vi "Manual control operator action.vi"(6 "error in":errorcluster, 8 "Abort Test":T1, 9 "Motion Steps in":string[](array[string]), 11 "input cluster":T2={"AT glass position"={"Tag Name"="S060.PXI.Signals.PlltData.SN", "Network Path"="172.15.51.1,1,0", "use opc"=FALSE, "DataSocket Reference"={"CWDSLib._DCWDataSocket"=refnum, "CWDSLib._DCWData"=refnum, "OnDataUpdated"=0, "OnStatusUpdated"=0}}, "AT shade position"={"Tag Name"="S060.PXI.Signals.PlltData.SN", "Network Path"="172.15.51.1,1,0", "use opc"=FALSE, "DataSocket Reference"={"CWDSLib._DCWDataSocket"=refnum, "CWDSLib._DCWData"=refnum, "OnDataUpdated"=0, "OnStatusUpdated"=0}}, "AT in glass wand lower pos"={"Tag Name"="S060.PXI.Signals.PlltData.SN", "Network Path"="172.15.51.1,1,0", "use opc"=FALSE, "DataSocket Reference"={"CWDSLib._DCWDataSocket"=refnum, "CWDSLib._DCWData"=refnum, "OnDataUpdated"=0, "OnStatusUpdated"=0}}, "AT in glass wand up pos"={"Tag Name"="S060.PXI.Signals.PlltData.SN", "Network Path"="172.15.51.1,1,0", "use opc"=FALSE, "DataSocket Reference"={"CWDSLib._DCWDataSocket"=refnum, "CWDSLib._DCWData"=refnum, "OnDataUpdated"=0, "OnStatusUpdated"=0}}, "AT in sunshad wand lower pos"={"Tag Name"="S060.PXI.Signals.PlltData.SN", "Network Path"="172.15.51.1,1,0", "use opc"=FALSE, "DataSocket Reference"={"CWDSLib._DCWDataSocket"=refnum, "CWDSLib._DCWData"=refnum, "OnDataUpdated"=0, "OnStatusUpdated"=0}}, "AT in sunshad wand up pos"={"Tag Name"="S060.PXI.Signals.PlltData.SN", "Network Path"="172.15.51.1,1,0", "use opc"=FALSE, "DataSocket Reference"={"CWDSLib._DCWDataSocket"=refnum, "CWDSLib._DCWData"=refnum, "OnDataUpdated"=0, "OnStatusUpdated"=0}}, "AT in wand home pos"={"Tag Name"="S060.PXI.Signals.PlltData.SN", "Network Path"="172.15.51.1,1,0", "use opc"=FALSE, "DataSocket Reference"={"CWDSLib._DCWDataSocket"=refnum, "CWDSLib._DCWData"=refnum, "OnDataUpdated"=0, "OnStatusUpdated"=0}}, "LVDT's Extended"={"Tag Name"="S060.PXI.Signals.PlltData.SN", "Network Path"="172.15.51.1,1,0", "use opc"=FALSE, "DataSocket Reference"={"CWDSLib._DCWDataSocket"=refnum, "CWDSLib._DCWData"=refnum, "OnDataUpdated"=0, "OnStatusUpdated"=0}}, "bolt check 1"={"Tag Name"="S060.PXI.Signals.PlltData.SN", "Network Path"="172.15.51.1,1,0", "use opc"=FALSE, "DataSocket Reference"={"CWDSLib._DCWDataSocket"=refnum, "CWDSLib._DCWData"=refnum, "OnDataUpdated"=0, "OnStatusUpdated"=0}}, "bolt check 2"={"Tag Name"="S060.PXI.Signals.PlltData.SN", "Network Path"="172.15.51.1,1,0", "use opc"=FALSE, "DataSocket Reference"={"CWDSLib._DCWDataSocket"=refnum, "CWDSLib._DCWData"=refnum, "OnDataUpdated"=0, "OnStatusUpdated"=0}}, "bolt check 3"={"Tag Name"="S060.PXI.Signals.PlltData.SN", "Network Path"="172.15.51.1,1,0", "use opc"=FALSE, "DataSocket Reference"={"CWDSLib._DCWDataSocket"=refnum, "CWDSLib._DCWData"=refnum, "OnDataUpdated"=0, "OnStatusUpdated"=0}}, "bolt check 4"={"Tag Name"="S060.PXI.Signals.PlltData.SN", "Network Path"="172.15.51.1,1,0", "use opc"=FALSE, "DataSocket Reference"={"CWDSLib._DCWDataSocket"=refnum, "CWDSLib._DCWData"=refnum, "OnDataUpdated"=0, "OnStatusUpdated"=0}}, "bolt check 5"={"Tag Name"="S060.PXI.Signals.PlltData.SN", "Network Path"="172.15.51.1,1,0", "use opc"=FALSE, "DataSocket Reference"={"CWDSLib._DCWDataSocket"=refnum, "CWDSLib._DCWData"=refnum, "OnDataUpdated"=0, "OnStatusUpdated"=0}}, "bolt check 6"={"Tag Name"="S060.PXI.Signals.PlltData.SN", "Network Path"="172.15.51.1,1,0", "use opc"=FALSE, "DataSocket Reference"={"CWDSLib._DCWDataSocket"=refnum, "CWDSLib._DCWData"=refnum, "OnDataUpdated"=0, "OnStatusUpdated"=0}}, "bolt check 7"={"Tag Name"="S060.PXI.Signals.PlltData.SN", "Network Path"="172.15.51.1,1,0", "use opc"=FALSE, "DataSocket Reference"={"CWDSLib._DCWDataSocket"=refnum, "CWDSLib._DCWData"=refnum, "OnDataUpdated"=0, "OnStatusUpdated"=0}}, "bolt check 8"={"Tag Name"="S060.PXI.Signals.PlltData.SN", "Network Path"="172.15.51.1,1,0", "use opc"=FALSE, "DataSocket Reference"={"CWDSLib._DCWDataSocket"=refnum, "CWDSLib._DCWData"=refnum, "OnDataUpdated"=0, "OnStatusUpdated"=0}}, "start"={"Tag Name"="S060.PXI.Signals.PlltData.SN", "Network Path"="172.15.51.1,1,0", "use opc"=FALSE, "DataSocket Reference"={"CWDSLib._DCWDataSocket"=refnum, "CWDSLib._DCWData"=refnum, "OnDataUpdated"=0, "OnStatusUpdated"=0}}, "abort"={"Tag Name"="S060.PXI.Signals.PlltData.SN", "Network Path"="172.15.51.1,1,0", "use opc"=FALSE, "DataSocket Reference"={"CWDSLib._DCWDataSocket"=refnum, "CWDSLib._DCWData"=refnum, "OnDataUpdated"=0, "OnStatusUpdated"=0}}, "LVDT's Retracted"={"Tag Name"="S060.PXI.Signals.PlltData.SN", "Network Path"="172.15.51.1,1,0", "use opc"=FALSE, "DataSocket Reference"={"CWDSLib._DCWDataSocket"=refnum, "CWDSLib._DCWData"=refnum, "OnDataUpdated"=0, "OnStatusUpdated"=0}}, "manual barcode print"={"Tag Name"="S060.PXI.Signals.PlltData.SN", "Network Path"="172.15.51.1,1,0", "use opc"=FALSE, "DataSocket Reference"={"CWDSLib._DCWDataSocket"=refnum, "CWDSLib._DCWData"=refnum, "OnDataUpdated"=0, "OnStatusUpdated"=0}}, "ss servo at open"={"Tag Name"="S060.PXI.Signals.PlltData.SN", "Network Path"="172.15.51.1,1,0", "use opc"=FALSE, "DataSocket Reference"={"CWDSLib._DCWDataSocket"=refnum, "CWDSLib._DCWData"=refnum, "OnDataUpdated"=0, "OnStatusUpdated"=0}}, "ss servo at close"={"Tag Name"="S060.PXI.Signals.PlltData.SN", "Network Path"="172.15.51.1,1,0", "use opc"=FALSE, "DataSocket Reference"={"CWDSLib._DCWDataSocket"=refnum, "CWDSLib._DCWData"=refnum, "OnDataUpdated"=0, "OnStatusUpdated"=0}}, "ss servo opening"={"Tag Name"="S060.PXI.Signals.PlltData.SN", "Network Path"="172.15.51.1,1,0", "use opc"=FALSE, "DataSocket Reference"={"CWDSLib._DCWDataSocket"=refnum, "CWDSLib._DCWData"=refnum, "OnDataUpdated"=0, "OnStatusUpdated"=0}}, "ss servo closing"={"Tag Name"="S060.PXI.Signals.PlltData.SN", "Network Path"="172.15.51.1,1,0", "use opc"=FALSE, "DataSocket Reference"={"CWDSLib._DCWDataSocket"=refnum, "CWDSLib._DCWData"=refnum, "OnDataUpdated"=0, "OnStatusUpdated"=0}}, "control slide at home"={"Tag Name"="S060.PXI.Signals.PlltData.SN", "Network Path"="172.15.51.1,1,0", "use opc"=FALSE, "DataSocket Reference"={"CWDSLib._DCWDataSocket"=refnum, "CWDSLib._DCWData"=refnum, "OnDataUpdated"=0, "OnStatusUpdated"=0}}, "control slide left good"={"Tag Name"="S060.PXI.Signals.PlltData.SN", "Network Path"="172.15.51.1,1,0", "use opc"=FALSE, "DataSocket Reference"={"CWDSLib._DCWDataSocket"=refnum, "CWDSLib._DCWData"=refnum, "OnDataUpdated"=0, "OnStatusUpdated"=0}}, "control slide left over stroke"={"Tag Name"="S060.PXI.Signals.PlltData.SN", "Network Path"="172.15.51.1,1,0", "use opc"=FALSE, "DataSocket Reference"={"CWDSLib._DCWDataSocket"=refnum, "CWDSLib._DCWData"=refnum, "OnDataUpdated"=0, "OnStatusUpdated"=0}}, "control slide right good"={"Tag Name"="S060.PXI.Signals.PlltData.SN", "Network Path"="172.15.51.1,1,0", "use opc"=FALSE, "DataSocket Reference"={"CWDSLib._DCWDataSocket"=refnum, "CWDSLib._DCWData"=refnum, "OnDataUpdated"=0, "OnStatusUpdated"=0}}, "control slide right over stroke"={"Tag Name"="S060.PXI.Signals.PlltData.SN", "Network Path"="172.15.51.1,1,0", "use opc"=FALSE, "DataSocket Reference"={"CWDSLib._DCWDataSocket"=refnum, "CWDSLib._DCWData"=refnum, "OnDataUpdated"=0, "OnStatusUpdated"=0}}, "wind deflector high speed pos"={"Tag Name"="S060.PXI.Signals.PlltData.SN", "Network Path"="172.15.51.1,1,0", "use opc"=FALSE, "DataSocket Reference"={"CWDSLib._DCWDataSocket"=refnum, "CWDSLib._DCWData"=refnum, "OnDataUpdated"=0, "OnStatusUpdated"=0}}, "wind deflector low speed pos"={"Tag Name"="S060.PXI.Signals.PlltData.SN", "Network Path"="172.15.51.1,1,0", "use opc"=FALSE, "DataSocket Reference"={"CWDSLib._DCWDataSocket"=refnum, "CWDSLib._DCWData"=refnum, "OnDataUpdated"=0, "OnStatusUpdated"=0}}, "AT VentPMACatHome"={"Tag Name"="S060.PXI.Signals.PlltData.SN", "Network Path"="172.15.51.1,1,0", "use opc"=FALSE, "DataSocket Reference"={"CWDSLib._DCWDataSocket"=refnum, "CWDSLib._DCWData"=refnum, "OnDataUpdated"=0, "OnStatusUpdated"=0}}, "AT VentPMACisExtend"={"Tag Name"="S060.PXI.Signals.PlltData.SN", "Network Path"="172.15.51.1,1,0", "use opc"=FALSE, "DataSocket Reference"={"CWDSLib._DCWDataSocket"=refnum, "CWDSLib._DCWData"=refnum, "OnDataUpdated"=0, "OnStatusUpdated"=0}}, "SS Barcode Scanner Bypassed"={"Tag Name"="S060.PXI.Signals.PlltData.SN", "Network Path"="172.15.51.1,1,0", "use opc"=FALSE, "DataSocket Reference"={"CWDSLib._DCWDataSocket"=refnum, "CWDSLib._DCWData"=refnum, "OnDataUpdated"=0, "OnStatusUpdated"=0}}, "Check Frame Barcode"={"Tag Name"="S060.PXI.Signals.PlltData.SN", "Network Path"="172.15.51.1,1,0", "use opc"=FALSE, "DataSocket Reference"={"CWDSLib._DCWDataSocket"=refnum, "CWDSLib._DCWData"=refnum, "OnDataUpdated"=0, "OnStatusUpdated"=0}}, "Z LVDTs Extended"={"Tag Name"="S060.PXI.Signals.PlltData.SN", "Network Path"="172.15.51.1,1,0", "use opc"=FALSE, "DataSocket Reference"={"CWDSLib._DCWDataSocket"=refnum, "CWDSLib._DCWData"=refnum, "OnDataUpdated"=0, "OnStatusUpdated"=0}}, "NVH Operator Pass"={"Tag Name"="S060.PXI.Signals.PlltData.SN", "Network Path"="172.15.51.1,1,0", "use opc"=FALSE, "DataSocket Reference"={"CWDSLib._DCWDataSocket"=refnum, "CWDSLib._DCWData"=refnum, "OnDataUpdated"=0, "OnStatusUpdated"=0}}, "NVH Operator Fail"={"Tag Name"="S060.PXI.Signals.PlltData.SN", "Network Path"="172.15.51.1,1,0", "use opc"=FALSE, "DataSocket Reference"={"CWDSLib._DCWDataSocket"=refnum, "CWDSLib._DCWData"=refnum, "OnDataUpdated"=0, "OnStatusUpdated"=0}}, "NVH Operator Express Glass Open"={"Tag Name"="S060.PXI.Signals.PlltData.SN", "Network Path"="172.15.51.1,1,0", "use opc"=FALSE, "DataSocket Reference"={"CWDSLib._DCWDataSocket"=refnum, "CWDSLib._DCWData"=refnum, "OnDataUpdated"=0, "OnStatusUpdated"=0}}, "NVH Operator Express Glass Close"={"Tag Name"="S060.PXI.Signals.PlltData.SN", "Network Path"="172.15.51.1,1,0", "use opc"=FALSE, "DataSocket Reference"={"CWDSLib._DCWDataSocket"=refnum, "CWDSLib._DCWData"=refnum, "OnDataUpdated"=0, "OnStatusUpdated"=0}}, "NVH Operator Express Rollo Open01"={"Tag Name"="S060.PXI.Signals.PlltData.SN", "Network Path"="172.15.51.1,1,0", "use opc"=FALSE, "DataSocket Reference"={"CWDSLib._DCWDataSocket"=refnum, "CWDSLib._DCWData"=refnum, "OnDataUpdated"=0, "OnStatusUpdated"=0}}, "NVH Operator Express Rollo Close01"={"Tag Name"="S060.PXI.Signals.PlltData.SN", "Network Path"="172.15.51.1,1,0", "use opc"=FALSE, "DataSocket Reference"={"CWDSLib._DCWDataSocket"=refnum, "CWDSLib._DCWData"=refnum, "OnDataUpdated"=0, "OnStatusUpdated"=0}}, "NVH Operator Express Rollo Open02"={"Tag Name"="S060.PXI.Signals.PlltData.SN", "Network Path"="172.15.51.1,1,0", "use opc"=FALSE, "DataSocket Reference"={"CWDSLib._DCWDataSocket"=refnum, "CWDSLib._DCWData"=refnum, "OnDataUpdated"=0, "OnStatusUpdated"=0}}, "NVH Operator Express Rollo Close02"={"Tag Name"="S060.PXI.Signals.PlltData.SN", "Network Path"="172.15.51.1,1,0", "use opc"=FALSE, "DataSocket Reference"={"CWDSLib._DCWDataSocket"=refnum, "CWDSLib._DCWData"=refnum, "OnDataUpdated"=0, "OnStatusUpdated"=0}}, "NVH Operator Vent Open Noise"={"Tag Name"="S060.PXI.Signals.PlltData.SN", "Network Path"="172.15.51.1,1,0", "use opc"=FALSE, "DataSocket Reference"={"CWDSLib._DCWDataSocket"=refnum, "CWDSLib._DCWData"=refnum, "OnDataUpdated"=0, "OnStatusUpdated"=0}}, "NVH Operator Vent Close Noise"={"Tag Name"="S060.PXI.Signals.PlltData.SN", "Network Path"="172.15.51.1,1,0", "use opc"=FALSE, "DataSocket Reference"={"CWDSLib._DCWDataSocket"=refnum, "CWDSLib._DCWData"=refnum, "OnDataUpdated"=0, "OnStatusUpdated"=0}}, "NVH Operator Sunshade Open Noise"={"Tag Name"="S060.PXI.Signals.PlltData.SN", "Network Path"="172.15.51.1,1,0", "use opc"=FALSE, "DataSocket Reference"={"CWDSLib._DCWDataSocket"=refnum, "CWDSLib._DCWData"=refnum, "OnDataUpdated"=0, "OnStatusUpdated"=0}}, "NVH Operator Sunshade Close Noise"={"Tag Name"="S060.PXI.Signals.PlltData.SN", "Network Path"="172.15.51.1,1,0", "use opc"=FALSE, "DataSocket Reference"={"CWDSLib._DCWDataSocket"=refnum, "CWDSLib._DCWData"=refnum, "OnDataUpdated"=0, "OnStatusUpdated"=0}}, "NVH Operator Glass Open Noise"={"Tag Name"="S060.PXI.Signals.PlltData.SN", "Network Path"="172.15.51.1,1,0", "use opc"=FALSE, "DataSocket Reference"={"CWDSLib._DCWDataSocket"=refnum, "CWDSLib._DCWData"=refnum, "OnDataUpdated"=0, "OnStatusUpdated"=0}}, "NVH Operator Glass Close Noise"={"Tag Name"="S060.PXI.Signals.PlltData.SN", "Network Path"="172.15.51.1,1,0", "use opc"=FALSE, "DataSocket Reference"={"CWDSLib._DCWDataSocket"=refnum, "CWDSLib._DCWData"=refnum, "OnDataUpdated"=0, "OnStatusUpdated"=0}}, "NVH Operator Finish"={"Tag Name"="S060.PXI.Signals.PlltData.SN", "Network Path"="172.15.51.1,1,0", "use opc"=FALSE, "DataSocket Reference"={"CWDSLib._DCWDataSocket"=refnum, "CWDSLib._DCWData"=refnum, "OnDataUpdated"=0, "OnStatusUpdated"=0}}, "NVH Operator Check"={"Tag Name"="S060.PXI.Signals.PlltData.SN", "Network Path"="172.15.51.1,1,0", "use opc"=FALSE, "DataSocket Reference"={"CWDSLib._DCWDataSocket"=refnum, "CWDSLib._DCWData"=refnum, "OnDataUpdated"=0, "OnStatusUpdated"=0}}, "windproof position"={"Tag Name"="S060.PXI.Signals.PlltData.SN", "Network Path"="172.15.51.1,1,0", "use opc"=FALSE, "DataSocket Reference"={"CWDSLib._DCWDataSocket"=refnum, "CWDSLib._DCWData"=refnum, "OnDataUpdated"=0, "OnStatusUpdated"=0}}, "NVH Operator Express Glass vent Open"={"Tag Name"="S060.PXI.Signals.PlltData.SN", "Network Path"="172.15.51.1,1,0", "use opc"=FALSE, "DataSocket Reference"={"CWDSLib._DCWDataSocket"=refnum, "CWDSLib._DCWData"=refnum, "OnDataUpdated"=0, "OnStatusUpdated"=0}}, "NVH Operator Express Glass Vent Close"={"Tag Name"="S060.PXI.Signals.PlltData.SN", "Network Path"="172.15.51.1,1,0", "use opc"=FALSE, "DataSocket Reference"={"CWDSLib._DCWDataSocket"=refnum, "CWDSLib._DCWData"=refnum, "OnDataUpdated"=0, "OnStatusUpdated"=0}}, "NVH Operator Re-do"={"Tag Name"="S060.PXI.Signals.PlltData.SN", "Network Path"="172.15.51.1,1,0", "use opc"=FALSE, "DataSocket Reference"={"CWDSLib._DCWDataSocket"=refnum, "CWDSLib._DCWData"=refnum, "OnDataUpdated"=0, "OnStatusUpdated"=0}}, "AT at vent ATS test pos"={"Tag Name"="S060.PXI.Signals.PlltData.SN", "Network Path"="172.15.51.1,1,0", "use opc"=FALSE, "DataSocket Reference"={"CWDSLib._DCWDataSocket"=refnum, "CWDSLib._DCWData"=refnum, "OnDataUpdated"=0, "OnStatusUpdated"=0}}, "AT at vent ATS Home pos"={"Tag Name"="S060.PXI.Signals.PlltData.SN", "Network Path"="172.15.51.1,1,0", "use opc"=FALSE, "DataSocket Reference"={"CWDSLib._DCWDataSocket"=refnum, "CWDSLib._DCWData"=refnum, "OnDataUpdated"=0, "OnStatusUpdated"=0}}, "Start Adjust LVDT"={"Tag Name"="S060.PXI.Signals.PlltData.SN", "Network Path"="172.15.51.1,1,0", "use opc"=FALSE, "DataSocket Reference"={"CWDSLib._DCWDataSocket"=refnum, "CWDSLib._DCWData"=refnum, "OnDataUpdated"=0, "OnStatusUpdated"=0}}, "Finish Adjust LVDT"={"Tag Name"="S060.PXI.Signals.PlltData.SN", "Network Path"="172.15.51.1,1,0", "use opc"=FALSE, "DataSocket Reference"={"CWDSLib._DCWDataSocket"=refnum, "CWDSLib._DCWData"=refnum, "OnDataUpdated"=0, "OnStatusUpdated"=0}}} {"AT in sunshad wand up pos"."DataSocket Reference"."OnStatusUpdated" format="%.0x"; "AT in sunshad wand up pos"."DataSocket Reference"."OnDataUpdated" format="%.0x"; "AT in glass wand up pos"."DataSocket Reference"."OnStatusUpdated" format="%.0x"; "AT in glass wand up pos"."DataSocket Reference"."OnDataUpdated" format="%.0x"; "Finish Adjust LVDT"."DataSocket Reference"."OnStatusUpdated" format="%.0x"; "Finish Adjust LVDT"."DataSocket Reference"."OnDataUpdated" format="%.0x"; "Start Adjust LVDT"."DataSocket Reference"."OnStatusUpdated" format="%.0x"; "Start Adjust LVDT"."DataSocket Reference"."OnDataUpdated" format="%.0x"; "AT at vent ATS Home pos"."DataSocket Reference"."OnStatusUpdated" format="%.0x"; "AT at vent ATS Home pos"."DataSocket Reference"."OnDataUpdated" format="%.0x"; "AT at vent ATS test pos"."DataSocket Reference"."OnStatusUpdated" format="%.0x"; "AT at vent ATS test pos"."DataSocket Reference"."OnDataUpdated" format="%.0x"; "NVH Operator Re-do"."DataSocket Reference"."OnStatusUpdated" format="%.0x"; "NVH Operator Re-do"."DataSocket Reference"."OnDataUpdated" format="%.0x"; "NVH Operator Express Glass Vent Close"."DataSocket Reference"."OnStatusUpdated" format="%.0x"; "NVH Operator Express Glass Vent Close"."DataSocket Reference"."OnDataUpdated" format="%.0x"; "NVH Operator Express Glass vent Open"."DataSocket Reference"."OnStatusUpdated" format="%.0x"; "NVH Operator Express Glass vent Open"."DataSocket Reference"."OnDataUpdated" format="%.0x"; "windproof position"."DataSocket Reference"."OnStatusUpdated" format="%.0x"; "windproof position"."DataSocket Reference"."OnDataUpdated" format="%.0x"; "NVH Operator Check"."DataSocket Reference"."OnStatusUpdated" format="%.0x"; "NVH Operator Check"."DataSocket Reference"."OnDataUpdated" format="%.0x"; "NVH Operator Finish"."DataSocket Reference"."OnStatusUpdated" format="%.0x"; "NVH Operator Finish"."DataSocket Reference"."OnDataUpdated" format="%.0x"; "NVH Operator Glass Close Noise"."DataSocket Reference"."OnStatusUpdated" format="%.0x"; "NVH Operator Glass Close Noise"."DataSocket Reference"."OnDataUpdated" format="%.0x"; "NVH Operator Glass Open Noise"."DataSocket Reference"."OnStatusUpdated" format="%.0x"; "NVH Operator Glass Open Noise"."DataSocket Reference"."OnDataUpdated" format="%.0x"; "NVH Operator Sunshade Close Noise"."DataSocket Reference"."OnStatusUpdated" format="%.0x"; "NVH Operator Sunshade Close Noise"."DataSocket Reference"."OnDataUpdated" format="%.0x"; "NVH Operator Sunshade Open Noise"."DataSocket Reference"."OnStatusUpdated" format="%.0x"; "NVH Operator Sunshade Open Noise"."DataSocket Reference"."OnDataUpdated" format="%.0x"; "NVH Operator Vent Close Noise"."DataSocket Reference"."OnStatusUpdated" format="%.0x"; "NVH Operator Vent Close Noise"."DataSocket Reference"."OnDataUpdated" format="%.0x"; "NVH Operator Vent Open Noise"."DataSocket Reference"."OnStatusUpdated" format="%.0x"; "NVH Operator Vent Open Noise"."DataSocket Reference"."OnDataUpdated" format="%.0x"; "NVH Operator Express Rollo Close02"."DataSocket Reference"."OnStatusUpdated" format="%.0x"; "NVH Operator Express Rollo Close02"."DataSocket Reference"."OnDataUpdated" format="%.0x"; "NVH Operator Express Rollo Open02"."DataSocket Reference"."OnStatusUpdated" format="%.0x"; "NVH Operator Express Rollo Open02"."DataSocket Reference"."OnDataUpdated" format="%.0x"; "NVH Operator Express Rollo Close01"."DataSocket Reference"."OnStatusUpdated" format="%.0x"; "NVH Operator Express Rollo Close01"."DataSocket Reference"."OnDataUpdated" format="%.0x"; "NVH Operator Express Rollo Open01"."DataSocket Reference"."OnStatusUpdated" format="%.0x"; "NVH Operator Express Rollo Open01"."DataSocket Reference"."OnDataUpdated" format="%.0x"; "NVH Operator Express Glass Close"."DataSocket Reference"."OnStatusUpdated" format="%.0x"; "NVH Operator Express Glass Close"."DataSocket Reference"."OnDataUpdated" format="%.0x"; "NVH Operator Express Glass Open"."DataSocket Reference"."OnStatusUpdated" format="%.0x"; "NVH Operator Express Glass Open"."DataSocket Reference"."OnDataUpdated" format="%.0x"; "NVH Operator Fail"."DataSocket Reference"."OnStatusUpdated" format="%.0x"; "NVH Operator Fail"."DataSocket Reference"."OnDataUpdated" format="%.0x"; "NVH Operator Pass"."DataSocket Reference"."OnStatusUpdated" format="%.0x"; "NVH Operator Pass"."DataSocket Reference"."OnDataUpdated" format="%.0x"; "Z LVDTs Extended"."DataSocket Reference"."OnStatusUpdated" format="%.0x"; "Z LVDTs Extended"."DataSocket Reference"."OnDataUpdated" format="%.0x"; "Check Frame Barcode"."DataSocket Reference"."OnStatusUpdated" format="%.0x"; "Check Frame Barcode"."DataSocket Reference"."OnDataUpdated" format="%.0x"; "SS Barcode Scanner Bypassed"."DataSocket Reference"."OnStatusUpdated" format="%.0x"; "SS Barcode Scanner Bypassed"."DataSocket Reference"."OnDataUpdated" format="%.0x"; "AT VentPMACisExtend"."DataSocket Reference"."OnStatusUpdated" format="%.0x"; "AT VentPMACisExtend"."DataSocket Reference"."OnDataUpdated" format="%.0x"; "AT VentPMACatHome"."DataSocket Reference"."OnStatusUpdated" format="%.0x"; "AT VentPMACatHome"."DataSocket Reference"."OnDataUpdated" format="%.0x"; "wind deflector low speed pos"."DataSocket Reference"."OnStatusUpdated" format="%.0x"; "wind deflector low speed pos"."DataSocket Reference"."OnDataUpdated" format="%.0x"; "wind deflector high speed pos"."DataSocket Reference"."OnStatusUpdated" format="%.0x"; "wind deflector high speed pos"."DataSocket Reference"."OnDataUpdated" format="%.0x"; "control slide right over stroke"."DataSocket Reference"."OnStatusUpdated" format="%.0x"; "control slide right over stroke"."DataSocket Reference"."OnDataUpdated" format="%.0x"; "control slide right good"."DataSocket Reference"."OnStatusUpdated" format="%.0x"; "control slide right good"."DataSocket Reference"."OnDataUpdated" format="%.0x"; "control slide left over stroke"."DataSocket Reference"."OnStatusUpdated" format="%.0x"; "control slide left over stroke"."DataSocket Reference"."OnDataUpdated" format="%.0x"; "control slide left good"."DataSocket Reference"."OnStatusUpdated" format="%.0x"; "control slide left good"."DataSocket Reference"."OnDataUpdated" format="%.0x"; "control slide at home"."DataSocket Reference"."OnStatusUpdated" format="%.0x"; "control slide at home"."DataSocket Reference"."OnDataUpdated" format="%.0x"; "ss servo closing"."DataSocket Reference"."OnStatusUpdated" format="%.0x"; "ss servo closing"."DataSocket Reference"."OnDataUpdated" format="%.0x"; "ss servo opening"."DataSocket Reference"."OnStatusUpdated" format="%.0x"; "ss servo opening"."DataSocket Reference"."OnDataUpdated" format="%.0x"; "ss servo at close"."DataSocket Reference"."OnStatusUpdated" format="%.0x"; "ss servo at close"."DataSocket Reference"."OnDataUpdated" format="%.0x"; "ss servo at open"."DataSocket Reference"."OnStatusUpdated" format="%.0x"; "ss servo at open"."DataSocket Reference"."OnDataUpdated" format="%.0x"; "manual barcode print"."DataSocket Reference"."OnStatusUpdated" format="%.0x"; "manual barcode print"."DataSocket Reference"."OnDataUpdated" format="%.0x"; "LVDT's Retracted"."DataSocket Reference"."OnStatusUpdated" format="%.0x"; "LVDT's Retracted"."DataSocket Reference"."OnDataUpdated" format="%.0x"; "abort"."DataSocket Reference"."OnStatusUpdated" format="%.0x"; "abort"."DataSocket Reference"."OnDataUpdated" format="%.0x"; "start"."DataSocket Reference"."OnStatusUpdated" format="%.0x"; "start"."DataSocket Reference"."OnDataUpdated" format="%.0x"; "bolt check 8"."DataSocket Reference"."OnStatusUpdated" format="%.0x"; "bolt check 8"."DataSocket Reference"."OnDataUpdated" format="%.0x"; "bolt check 7"."DataSocket Reference"."OnStatusUpdated" format="%.0x"; "bolt check 7"."DataSocket Reference"."OnDataUpdated" format="%.0x"; "bolt check 6"."DataSocket Reference"."OnStatusUpdated" format="%.0x"; "bolt check 6"."DataSocket Reference"."OnDataUpdated" format="%.0x"; "bolt check 5"."DataSocket Reference"."OnStatusUpdated" format="%.0x"; "bolt check 5"."DataSocket Reference"."OnDataUpdated" format="%.0x"; "bolt check 4"."DataSocket Reference"."OnStatusUpdated" format="%.0x"; "bolt check 4"."DataSocket Reference"."OnDataUpdated" format="%.0x"; "bolt check 3"."DataSocket Reference"."OnStatusUpdated" format="%.0x"; "bolt check 3"."DataSocket Reference"."OnDataUpdated" format="%.0x"; "bolt check 2"."DataSocket Reference"."OnStatusUpdated" format="%.0x"; "bolt check 2"."DataSocket Reference"."OnDataUpdated" format="%.0x"; "bolt check 1"."DataSocket Reference"."OnStatusUpdated" format="%.0x"; "bolt check 1"."DataSocket Reference"."OnDataUpdated" format="%.0x"; "LVDT's Extended"."DataSocket Reference"."OnStatusUpdated" format="%.0x"; "LVDT's Extended"."DataSocket Reference"."OnDataUpdated" format="%.0x"; "AT in wand home pos"."DataSocket Reference"."OnStatusUpdated" format="%.0x"; "AT in wand home pos"."DataSocket Reference"."OnDataUpdated" format="%.0x"; "AT in sunshad wand lower pos"."DataSocket Reference"."OnStatusUpdated" format="%.0x"; "AT in sunshad wand lower pos"."DataSocket Reference"."OnDataUpdated" format="%.0x"; "AT in glass wand lower pos"."DataSocket Reference"."OnStatusUpdated" format="%.0x"; "AT in glass wand lower pos"."DataSocket Reference"."OnDataUpdated" format="%.0x"; "AT shade position"."DataSocket Reference"."OnStatusUpdated" format="%.0x"; "AT shade position"."DataSocket Reference"."OnDataUpdated" format="%.0x"; "AT glass position"."DataSocket Reference"."OnStatusUpdated" format="%.0x"; "AT glass position"."DataSocket Reference"."OnDataUpdated" format="%.0x"}) -> (0 "error out":errorcluster, 1 "Step":string, 2 "data string":string, 3 "Motion Steps out":string[](array[string]))   [LabVIEW 2018]
uses:
  02.Type Def's/station plc read boolean tags.ctl
  05.UserVI's/type defs/plc path and tag.ctl
  <vilib>/Platform/dataskt.llb/DataSocket Reference Type.ctl
  05.UserVI's/type defs/EOL Global Digital Input Control.ctl
panel:
  # "start/abort only used by barcode instance, since there are discrete signals for this in the other stations."
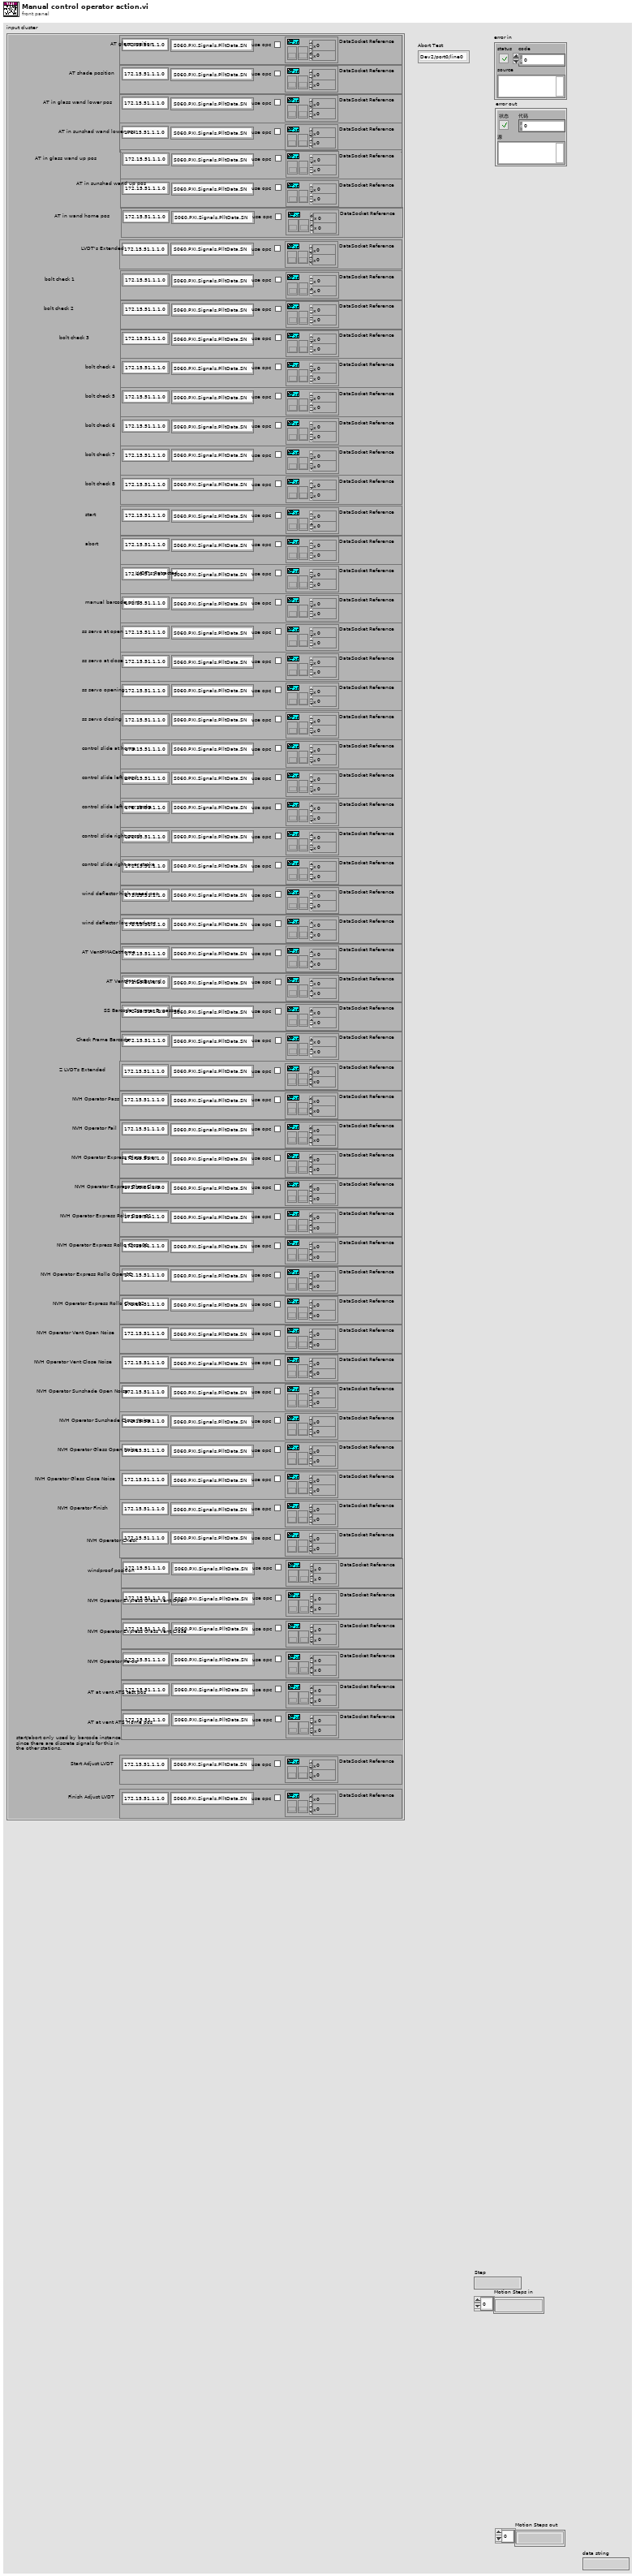
[diagram p1: front panel]
types:
  T1 = typedef "EOL Global Digital Input Control.ctl" = enum16{"Dev2/port0/line0", "Dev2/port0/line1", "Dev2/port0/line2", "Dev2/port0/line3", "Dev2/port0/line4", "Dev2/port0/line5", "Dev2/port0/line6", "Dev2/port0/line7", "Dev2/port1/line0", "Dev2/port1/line1", "Dev2/port1/line2", "Dev2/port1/line3", "Dev2/port1/line4", "Dev2/port1/line5", "Dev2/port1/line6", "Dev2/port1/line7", "Dev2/port2/line0", "Dev2/port2/line1", "Dev2/port2/line2", "Dev2/port2/line3", "Dev2/port2/line4", "Dev2/port2/line5", "Dev2/port2/line6", "Dev2/port2/line7", "Prerun Start Test", "Prerun Abort Test", "Audit Start Test", "Audit Abort Test", "Dev2/port3/line4", "Dev2/port3/line5", "Breakin Start Test", "Breakin Abort Test", "Not Implemented"}
  T2 = typedef "station plc read boolean tags.ctl" = cluster{"AT glass position":T3, "AT shade position":T3, "AT in glass wand lower pos":T3, "AT in glass wand up pos":T3, "AT in sunshad wand lower pos":T3, "AT in sunshad wand up pos":T3, "AT in wand home pos":T3, "LVDT's Extended":T3, "bolt check 1":T3, "bolt check 2":T3, "bolt check 3":T3, "bolt check 4":T3, "bolt check 5":T3, "bolt check 6":T3, "bolt check 7":T3, "bolt check 8":T3, "start":T3, "abort":T3, "LVDT's Retracted":T3, "manual barcode print":T3, "ss servo at open":T3, "ss servo at close":T3, "ss servo opening":T3, "ss servo closing":T3, "control slide at home":T3, "control slide left good":T3, "control slide left over stroke":T3, "control slide right good":T3, "control slide right over stroke":T3, "wind deflector high speed pos":T3, "wind deflector low speed pos":T3, "AT VentPMACatHome":T3, "AT VentPMACisExtend":T3, "SS Barcode Scanner Bypassed":T3, "Check Frame Barcode":T3, "Z LVDTs Extended":T3, "NVH Operator Pass":T3, "NVH Operator Fail":T3, "NVH Operator Express Glass Open":T3, "NVH Operator Express Glass Close":T3, "NVH Operator Express Rollo Open01":T3, "NVH Operator Express Rollo Close01":T3, "NVH Operator Express Rollo Open02":T3, "NVH Operator Express Rollo Close02":T3, "NVH Operator Vent Open Noise":T3, "NVH Operator Vent Close Noise":T3, "NVH Operator Sunshade Open Noise":T3, "NVH Operator Sunshade Close Noise":T3, "NVH Operator Glass Open Noise":T3, "NVH Operator Glass Close Noise":T3, "NVH Operator Finish":T3, "NVH Operator Check":T3, "windproof position":T3, "NVH Operator Express Glass vent Open":T3, "NVH Operator Express Glass Vent Close":T3, "NVH Operator Re-do":T3, "AT at vent ATS test pos":T3, "AT at vent ATS Home pos":T3, "Start Adjust LVDT":T3, "Finish Adjust LVDT":T3}
  T3 = typedef "plc path and tag.ctl" = cluster{"Tag Name":string, "Network Path":string, "use opc":bool, "DataSocket Reference":T4}
  T4 = typedef "DataSocket Reference Type.ctl" = cluster{"CWDSLib._DCWDataSocket":refnum<k7>, "CWDSLib._DCWData":refnum<k7>, "OnDataUpdated":u32, "OnStatusUpdated":u32}
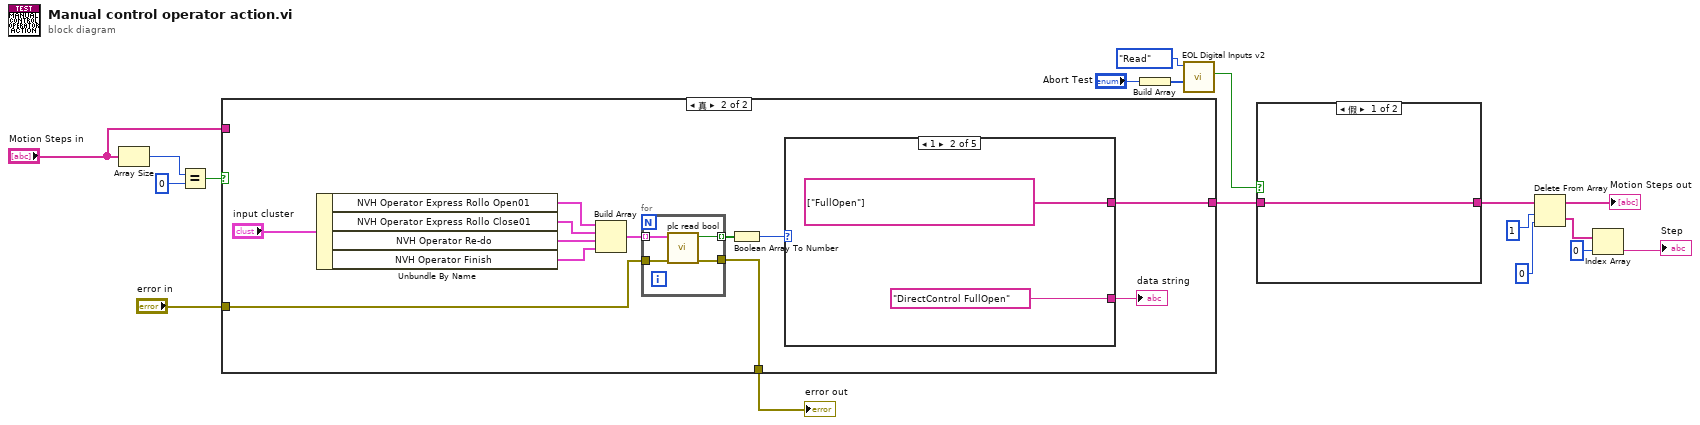
[diagram p0: block diagram]
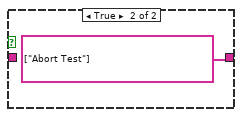
[diagram p2: hidden frame]
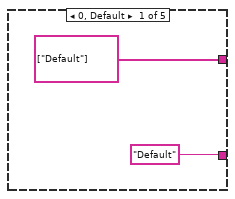
[diagram p4: hidden frame]
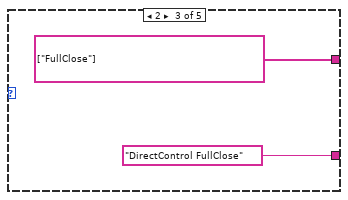
[diagram p5: hidden frame]
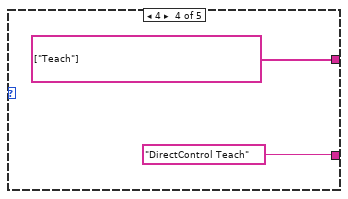
[diagram p6: hidden frame]
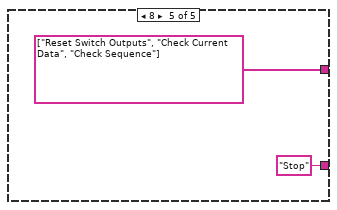
[diagram p7: hidden frame]
diagram:
  n1 = Array Size(array="Motion Steps in") -> (size(s)=w10:i32)
  n2 = Equal?(x=w10, y=0) -> (x = y?=w11:bool)
  n3 = case shown="真" w11 {
    tunnel: "Motion Steps in" -> [w20 _]
    tunnel: [w20 w25] -> w3
    tunnel: "error in" -> [w19 w22]
    tunnel: [w19 w21] -> w1
    frame False {
    }
    frame True {
      n4 = Unbundle By Name("input cluster") -> ("NVH Operator Express Rollo Open01"=w31:T3, "NVH Operator Express Rollo Close01"=w30:T3, "NVH Operator Re-do"=w26:T3, "NVH Operator Finish"=w24:T3)
      n5 = Build Array(w31, w30, w26, w24) -> (w29:T3[])
      n6 = for {
        tunnel: w29 -> [w46] mode=indexing
        tunnel: [w45] -> w28 mode=indexing
        tunnel: w22 -> [w44]
        tunnel: [w43] -> w21
        n7 = call "plc read bool.vi"("error in"=w44, "addr,tag"=w46) -> ("error out"=w43:errorcluster, "value"=w45:bool)  [unwired: 8 in]
      }
      n8 = Boolean Array To Number(Boolean array=w28) -> (number=w27:u32)
      n9 = case shown="1" w27 {
        tunnel: [string[] ["Default"] string[] ["FullOpen"] string[] ["FullClose"] string[] ["Teach"] string[] ["Reset Switch Outputs", "Check Current Data", "Check Sequence"]] -> w25
        tunnel: ["Default" "DirectControl FullOpen" "DirectControl FullClose" "DirectControl Teach" "Stop"] -> w23
        frame 0, Default {
        }
        frame 1 {
        }
        frame 2 {
        }
        frame 4 {
        }
        frame 8 {
        }
      }
      "data string" <- w23
    }
  }
  "error out" <- w1
  n10 = Build Array("Abort Test") -> (w8:T1[])
  n11 = call "EOL Digital Inputs v2.vi"("Digital Inputs Array"=w8, "Mode"=enum16{"Init", "Read", "Read All", "Close"}."Read") -> ("Single Input"=w5:bool)  [unwired: 7 in, 2 out]
  n12 = case shown="假" w5 {
    tunnel: [w47 string[] ["Abort Test"]] -> w4
    tunnel: w3 -> [w47 _]
    frame False {
    }
    frame True {
    }
  }
  n13 = Delete From Array(array=w4, length=1, index=0) -> (deleted portion=w15:string[], array with subset deleted=→"Motion Steps out":string[])
  n14 = Index Array(array=w15, index=0) -> (element=→"Step":string)
